vi "Get Time Data Obj.vi"(0 "reference in":refnum<class "WaveFile.lvclass">, 5 "error in (no error)":errorcluster) -> (14 "reference out":refnum<class "WaveFile.lvclass">, 16 "Time data ref":refnum<class "GSwFormDSP.lvclass">, 19 "error out":errorcluster)   [LabVIEW 2020, in "WaveFile.lvclass"]
uses:
  WaveFile.lvclass
  API/GSwFormDSP_class/GSwFormDSP.lvclass
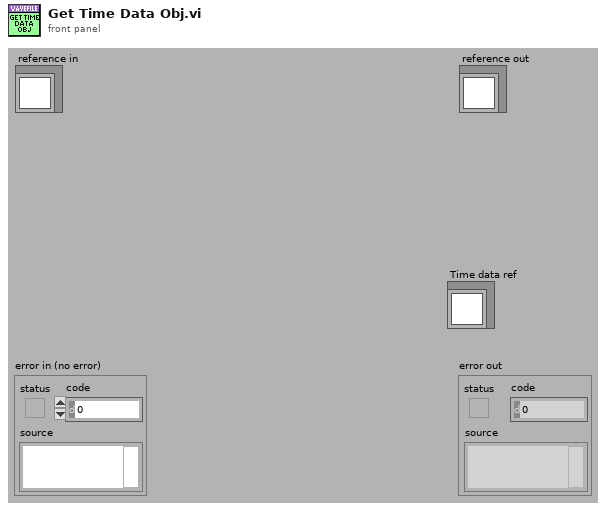
[diagram p1: front panel]
types:
  T1 = typedef "WaveFile.lvclass/ObjectAttributes.ctl" = cluster{"Time Data":refnum<class "GSwFormDSP.lvclass">, "New Time Data Obj?":bool, "NIST File Header":T2}
  T2 = typedef "WaveFile.lvclass/NIST File Header.ctl" = cluster{"Version":string, "Header Nb Bytes":i32, "Nb Samples":i32, "Nb Bytes/sample":i32, "Nb Channels":i32, "byte order":enum16{"big-endian, network order", "native, host order", "little-endian"}, "Fs":dbl, "Valid Header?":bool}
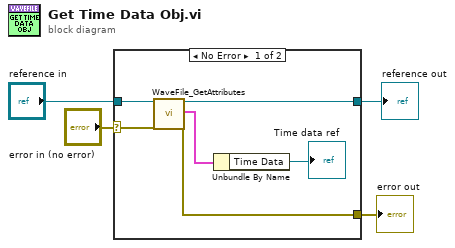
[diagram p0: block diagram]
diagram:
  n1 = case shown="No Error" "error in (no error)" {
    selector: "error in (no error)" -> [w10 w12]
    tunnel: [w6 w12] -> w3
    tunnel: [w9 w11] -> w1
    tunnel: "reference in" -> [w7 w11]
    frame No Error {
      n2 = call "WaveFile_GetAttributes.vi"("reference in"=w7, "error in (no error)"=w10) -> ("reference out"=w9:refnum<class "WaveFile.lvclass">, "attributes"=w8:T1, "error out"=w6:errorcluster)  [unwired: 14 in, 1 out]
      n3 = Unbundle By Name(w8) -> ("Time Data"=→"Time data ref":refnum<class "GSwFormDSP.lvclass">)
    }
    frame Error {
    }
  }
  "error out" <- w3
  "reference out" <- w1
